vi "TstBldr_CloseProject.vi"(0 "Engine reference":refnum<k7>, 5 "Sequence File Ref":refnum<k7>, 7 "VeriStand version info":T1, 11 "error in":errorcluster, 12 "Sequence index":i32, 13 "Condition run?":bool=TRUE) -> (4 "Engine reference (out)":refnum<k7>, 6 "Sequence File Ref(out)":refnum<k7>, 8 "VeriStand version info (out)":T1, 14 "Sequence index out":i32, 15 "error out":errorcluster)   [LabVIEW 2010]
doc: "This VI creates the TestStand steps to stop the VeriStand (VS) workspace by closing the VS project"
uses:
  SeqBuilder/Ctls/dotNetAssemblyInfo.ctl
  SeqBuilder/Ctls/VSModuleTokens.ctl
  vs_StopProjectSteps.ctl
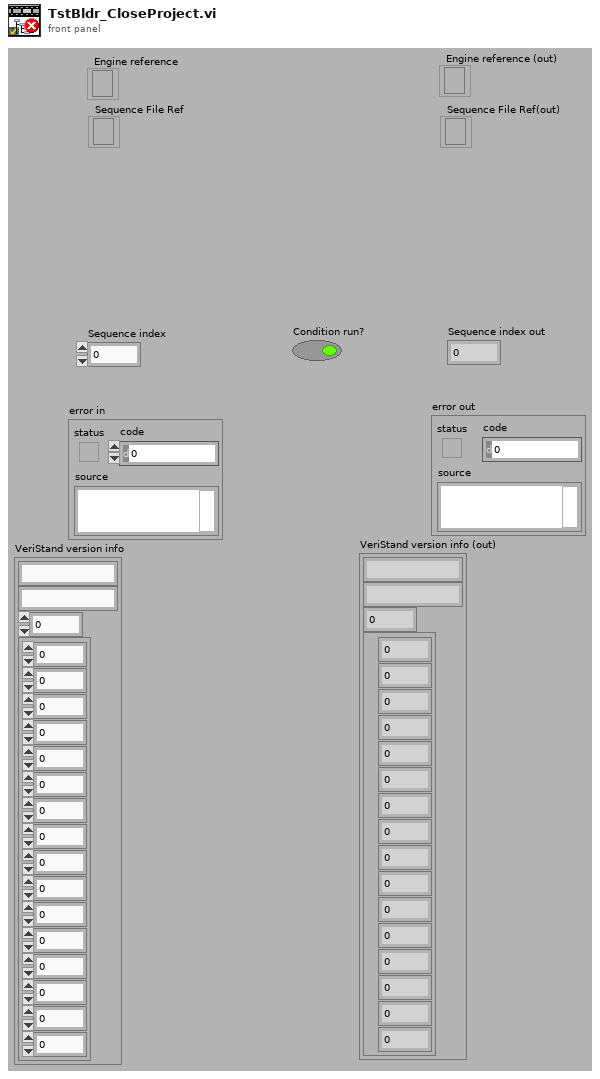
[diagram p1: front panel]
types:
  T1 = typedef "dotNetAssemblyInfo.ctl" = cluster{"VeriStand.exe Path":string, "Assembly":string, "Constructor Token":i32, "Module Token":T2}
  T2 = typedef "VSModuleTokens.ctl" = cluster{"GetIWorkspaceToken":i32, "GetIStimulusToken":i32, "GetIModelManagerToken":i32, "GetIProjectToken":i32, "RunProjectToken":i32, "CloseProjectToken":i32, "RunWorkspaceToken":i32, "StopWorkspaceToken":i32, "SetSingleChannelToken":i32, "SetMultipleParametersToken":i32, "RunStimulusToken":i32, "GetStimulusStateToken":i32, "Open WorkspaceToken":i32, "DeployToken":i32, "UndeployToken":i32, "QuitToken":i32}
  T3 = typedef "vs_StopProjectSteps.ctl" = enum16{"Undeploy", "Close Project", "Quit Loop"}
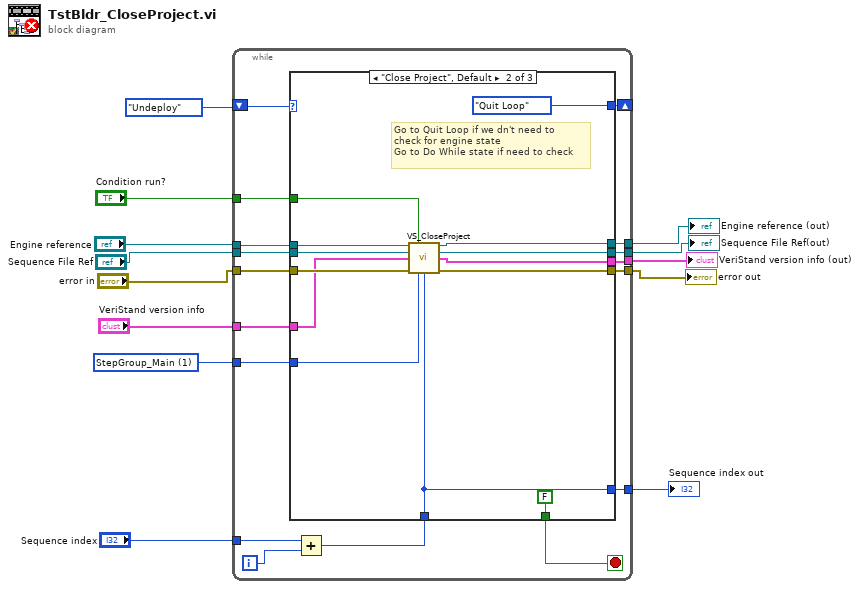
[diagram p0: block diagram]
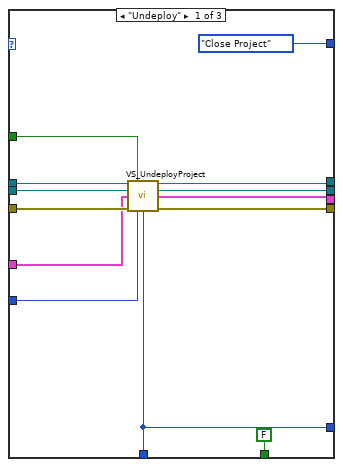
[diagram p2: hidden frame]
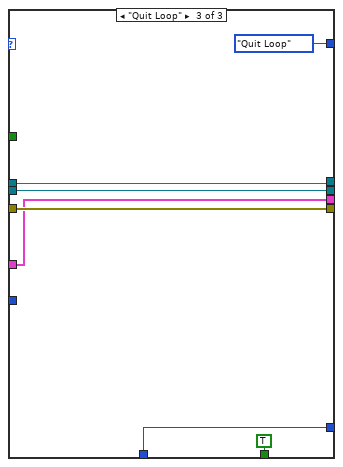
[diagram p3: hidden frame]
diagram:
  w3 = 1 items=["StepGroup_Setup", "StepGroup_Main", "StepGroup_Cleanup"] ("Step Group")
  n1 = while {
    shift-right: [w29] -> _
    shift-left: vs_StopProjectSteps."Undeploy" ("Enum") -> [w30]
    tunnel: "Engine reference" -> [w28]
    tunnel: "Sequence File Ref" -> [w27]
    tunnel: "error in" -> [w26]
    tunnel: "VeriStand version info" -> [w25]
    tunnel: [w24] -> w8
    tunnel: [w23] -> w6
    tunnel: [w22] -> w7
    tunnel: [w21] -> w5
    tunnel: "Condition run?" -> [w20]
    tunnel: w3 -> [w19]
    tunnel: "Sequence index" -> [w18]
    tunnel: [w15] -> w1
    i -> [w17]
    stop <- w14 stop-if-true
    n2 = Add(x=w18, y=w17) -> (x+y=w16:i32)
    n3 = case shown="\"Close Project\", Default" w30 {
      tunnel: [vs_StopProjectSteps."Close Project" ("Enum") vs_StopProjectSteps."Quit Loop" ("Enum") vs_StopProjectSteps."Quit Loop" ("Enum")] -> w29
      tunnel: w28 -> [w37 w55 w63]
      tunnel: w27 -> [w36 w54 w62]
      tunnel: w26 -> [w39 w53 w59]
      tunnel: w25 -> [w33 w52 w58]
      tunnel: [w38 w51 w59] -> w24
      tunnel: [w34 w50 w62] -> w23
      tunnel: [w32 w49 w58] -> w22
      tunnel: [w35 w48 w63] -> w21
      tunnel: w20 -> [w31 w47 _]
      tunnel: w19 -> [w41 w46 _]
      tunnel: w16 -> [w40 w45 w60]
      tunnel: [w40 w45 w60] -> w15
      tunnel: [FALSE FALSE TRUE] -> w14
      frame "Undeploy" {
        n4 = call "VS_UndeployProject.vi"("Engine Reference(in)"=w37, "Condition Run?"=w31, "Sequence File Ref(in)"=w36, "VeriStand version info"=w33, "error in"=w39, "Step Group"=w41, "Step Index"=w40) -> ("Engine reference(out)"=w35:refnum<k7>, "Sequence File Ref(out)"=w34:refnum<k7>, "VeriStand version info (out)"=w32:T1, "error out"=w38:errorcluster)  [unwired: 5 in]
      }
      frame "Close Project", Default {
        # "Go to Quit Loop if we dn't need to\ncheck for engine state\nGo to Do While state if need to check"
        n5 = call "VS_CloseProject.vi"("Engine Reference(in)"=w55, "Condition Run?"=w47, "Sequence File Ref(in)"=w54, "VeriStand version info"=w52, "error in"=w53, "Step Group"=w46, "Step Index"=w45) -> ("Engine reference(out)"=w48:refnum<k7>, "Sequence File Ref(out)"=w50:refnum<k7>, "VeriStand version info (out)"=w49:T1, "error out"=w51:errorcluster)  [unwired: 5 in]
      }
      frame "Quit Loop" {
      }
    }
  }
  "Sequence File Ref(out)" <- w6
  "Engine reference (out)" <- w5
  "error out" <- w8
  "Sequence index out" <- w1
  "VeriStand version info (out)" <- w7
